vi "Publish MPReading.vi"(8 "error in (no error)":errorcluster, 11 "CS++DMM in":refnum<class "CS++DMM.lvclass">) -> (0 "error out":errorcluster, 3 "CS++DMM out":refnum<class "CS++DMM.lvclass">)   [LabVIEW 2016, in "CS++DMM.lvlib" / "CS++DMM.lvclass"]
doc: "Publish Multi-Point Reading to PV."
uses:
  CS++DMM.lvclass
  CSPP_Core/Classes/CS++ProcessVariables/ProcessVariable/PV.lvclass
  PV-Enum.ctl
  CS++DMM.lvclass/CS++DMM.ctl
  CSPP_Core/Classes/CS++ProcessVariables/ProcessVariable/PV.lvclass/PV.ctl
  CSPP_Core/Classes/CS++ProcessVariables/ProcessVariable/Write Data.vi
  CSPP_Core/Classes/CS++ProcessVariables/ProcessVariable/Write Timestamp.vi
  CSPP_Core/Classes/CS++ProcessVariables/ProcessVariable/Write Quality.vi
  CSPP_Core/Classes/CS++ProcessVariables/ProcessVariable/Write status.vi
  CSPP_Core/Classes/CS++ProcessVariables/PVConnection/PVConnection.lvclass
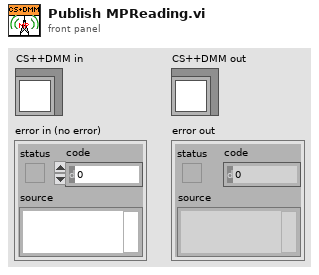
[diagram p1: front panel]
types:
  T1 = typedef "CS++DMM.lvlib/CS++DMM.lvclass/PV-Enum.ctl" = enum16{"AbsoluteResolution", "ACMaxFrequency", "ACMinFrequency", "ActualRange", "Alpha", "ApertureTime", "FixedReferenceJunction", "FrequencyVoltageRange", "PowerLineFrequency", "Range", "Reading", "Resistance", "SampleInterval", "TriggerDelay", "ApertureTimeUnit", "AutoZeroMode", "MeasCompleteDestination", "MeasurementFunction", "ReferenceJunctionType", "SampleCount", "SampleTrigger", "ThermocoupleType", "TransducerType", "TriggerCount", "TriggerSlope", "TriggerSource", "MPReading", "IsOverRange"}
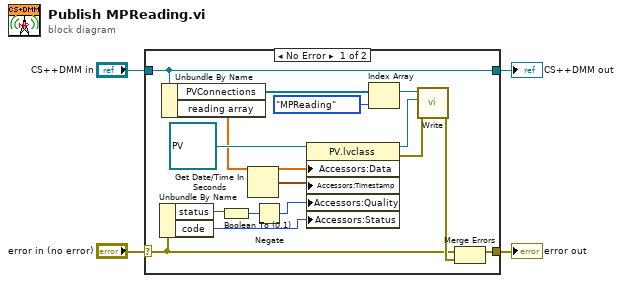
[diagram p0: block diagram]
diagram:
  n1 = case shown="No Error" "error in (no error)" {
    selector: "error in (no error)" -> [w8 w22]
    tunnel: [w7 w22] -> w3
    tunnel: [w11 w21] -> w1
    tunnel: "CS++DMM in" -> [w11 w21]
    frame No Error {
      n2 = Unbundle By Name(w8) -> ("status"=w16:bool, "code"=w13:i32)
      n3 = Unbundle By Name(w11) -> ("PVConnections"=w20:refnum<class "PVConnection.lvclass">[], "reading array"=w18:dbl[])
      n4 = Boolean To (0,1)(Boolean=w16) -> (0, 1=w15:i16)
      n5 = Get Date/Time In Seconds() -> (seconds since 1Jan1904=w17:timestamp)
      n6 = Negate(x=w15) -> (-x=w14:i16)
      n7 = property class="PV.lvclass"(reference=refnum<class "PV.lvclass"> refnum ("CS++ProcessVariables.lvlib:PV.lvclass"), "Accessors:Data"=w18, "Accessors:Timestamp"=w17, "Accessors:Quality"=w14, "Accessors:Status"=w13) -> (reference out=w12:refnum<class "PV.lvclass">, error out=w9:errorcluster)  [unwired: 1 in]
      n8 = Index Array(array=w20, index=PV-Enum."MPReading" ("PV-Enum")) -> (element=w6:refnum<class "PVConnection.lvclass">)
      n9 = call "Write.vi"("error in (no error)"=w9, "PV"=w12, "PVConnection in"=w6) -> ("error out"=w10:errorcluster)  [unwired: 7 in, 1 out]
      n10 = Merge Errors(w8, w10) -> (w7:errorcluster)
    }
    frame Error {
    }
  }
  "error out" <- w3
  "CS++DMM out" <- w1
